vi "Read Status Str Refnum.vi"(8 "error in (no error)":errorcluster, 11 "Tesla Factory Tester in":refnum<class "Tesla Factory Tester.lvclass">) -> (0 "error out":errorcluster, 2 "Status Str Refnum":refnum<vi>, 3 "Tesla Factory Tester out":refnum<class "Tesla Factory Tester.lvclass">)   [LabVIEW 2013, in "Tesla Factory Tester.lvlib" / "Tesla Factory Tester.lvclass"]
uses:
  Tesla Factory Tester.lvclass
  Tesla Factory Tester.lvclass/Tesla Factory Tester.ctl
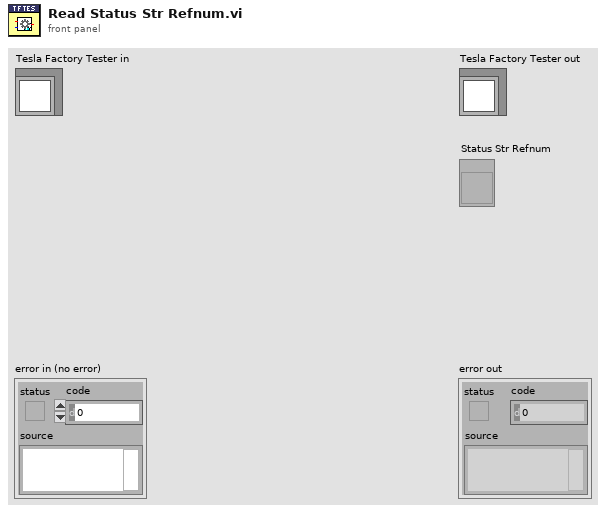
[diagram p1: front panel]
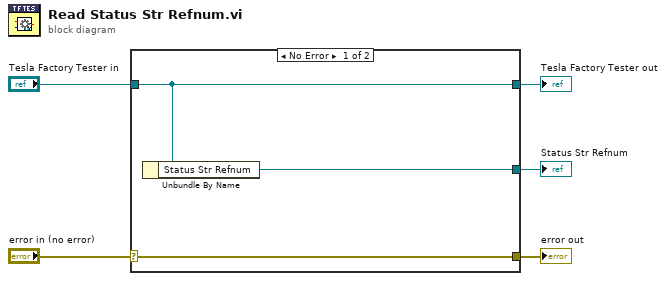
[diagram p0: block diagram]
diagram:
  n1 = case shown="No Error" "error in (no error)" {
    selector: "error in (no error)" -> [w8 w9]
    tunnel: [w8 w9] -> w4
    tunnel: [w7 w10] -> w2
    tunnel: "Tesla Factory Tester in" -> [w7 w10]
    tunnel: [w6 _] -> w1
    frame No Error {
      n2 = Unbundle By Name(w7) -> ("Status Str Refnum"=w6:refnum<vi>)
    }
    frame Error {
    }
  }
  "error out" <- w4
  "Tesla Factory Tester out" <- w2
  "Status Str Refnum" <- w1
